vi "Host Processing (SubVI).vi"(4 "Channel Data":cluster{"AI":T1, "DI":T5, "DO":T5, "Async":T8}={"AI"={"Interface"="AIO", "Interface Data"={"Command"="Configure", "SubCmd"="AI", "Data"=[{"Channel"="Mod1/ai0", "Min Value"=-5.0, "Max Value"=5.0, "Type"="Voltage", "Terminal Configure"=10083, "Dynamic"=0, "Dyn Type"="", "Data"=[], "File Name"="", "Column"=0, "Frequency"=0.0}, {"Channel"="Mod1/ai1", "Min Value"=-5.0, "Max Value"=5.0, "Type"="Voltage", "Terminal Configure"=10083, "Dynamic"=0, "Dyn Type"="", "Data"=[], "File Name"="", "Column"=0, "Frequency"=0.0}], "Timing"={"samples per channel"=4, "sample mode"=10123, "rate"=2.0}}}, "DI"={"Interface"="DIO", "Interface Data"={"Command"="Configure", "SubCmd"="DI", "Frequency"=20, "Data"=[{"Channel"="Mod2/port0/line0", "Data"=[], "Identification Name"=""}, {"Channel"="Mod2/port0/line1", "Data"=[], "Identification Name"=""}, {"Channel"="Mod2/port0/line2", "Data"=[], "Identification Name"=""}, {"Channel"="Mod2/port0/line3", "Data"=[], "Identification Name"=""}]}}, "DO"={"Interface"="DIO", "Interface Data"={"Command"="Configure", "SubCmd"="DO", "Frequency"=20, "Data"=[{"Channel"="Mod2/port0/line0", "Data"=[], "Identification Name"=""}, {"Channel"="Mod2/port0/line1", "Data"=[], "Identification Name"=""}, {"Channel"="Mod2/port0/line2", "Data"=[], "Identification Name"=""}, {"Channel"="Mod2/port0/line3", "Data"=[], "Identification Name"=""}]}}, "Async"={"Interface"="Async", "Interface Data"={"Command"="Configure", "SubCmd"="Async", "Data"=[{"Port"="com2", "Minor Frame Freq"=20, "Minor Frame Count"=1, "Frame Info"=[{"Frame ID"=1, "Message Info"=[{"Message"=[1, 2, 3, 4], "Message Name"="m1"}]}], "Sensor Type"=0, "OIM Address"=0}]}}} {"Async"."Interface Data"."Data"."Minor Frame Count" min=5 max=8 step=1; "AI"."Interface Data"."Timing"."sample mode" items=["Finite Samples"=10178, "Continuous Samples"=10123, "Hardware Timed Single Point"=12522]}, 5 "Serial Data":T13[](array[typedef]), 6 "Operation":T14(ring), 7 "DO Data":cluster{"Channel":string[], "Data":u8[]}={"Channel"=["Mod2/port1/line0", "Mod2/port1/line1", "Mod2/port1/line2", "Mod2/port1/line3"], "Data"=[0, 0, 0, 0]}, 8 "error in":errorcluster, 9 "connection ID in":refnum<k5>, 10 "queue in":refnum<queue>, 11 "IP":string) -> (0 "error out":errorcluster, 1 "connection ID":refnum<k5>, 2 "Queue out":refnum<queue>, 3 "data out":string)   [LabVIEW 2021]
uses:
  Async Serial/Controls/Async Message Info Cluster.ctl
  Async Serial/Controls/Async Update Cluster.ctl
  407f0374-129d-499a-9c6e-116d754379dc.vi
  Digital Output/SubVIs/Digital Dynamic Cluster.ctl
  Digital Output/Controls/DIO Interface Data.ctl
  Digital Output/Controls/DIO Configuration cluster.ctl
  Async Serial/Controls/Async Frame Info Cluster.ctl
  Async Serial/Controls/Async Serial Configuration Cluster.ctl
  Async Interface Data Cluster.ctl
  Async JSON Cluster.ctl
  Analog Output/Controls/AO Timing Cluster.ctl
  Analog Output/Controls/AO Channel Configuration Cluster.ctl
  Analog Output/Controls/AO Interface Data Cluster.ctl
  Analog Output/Controls/AO JSON Data Cluster.ctl
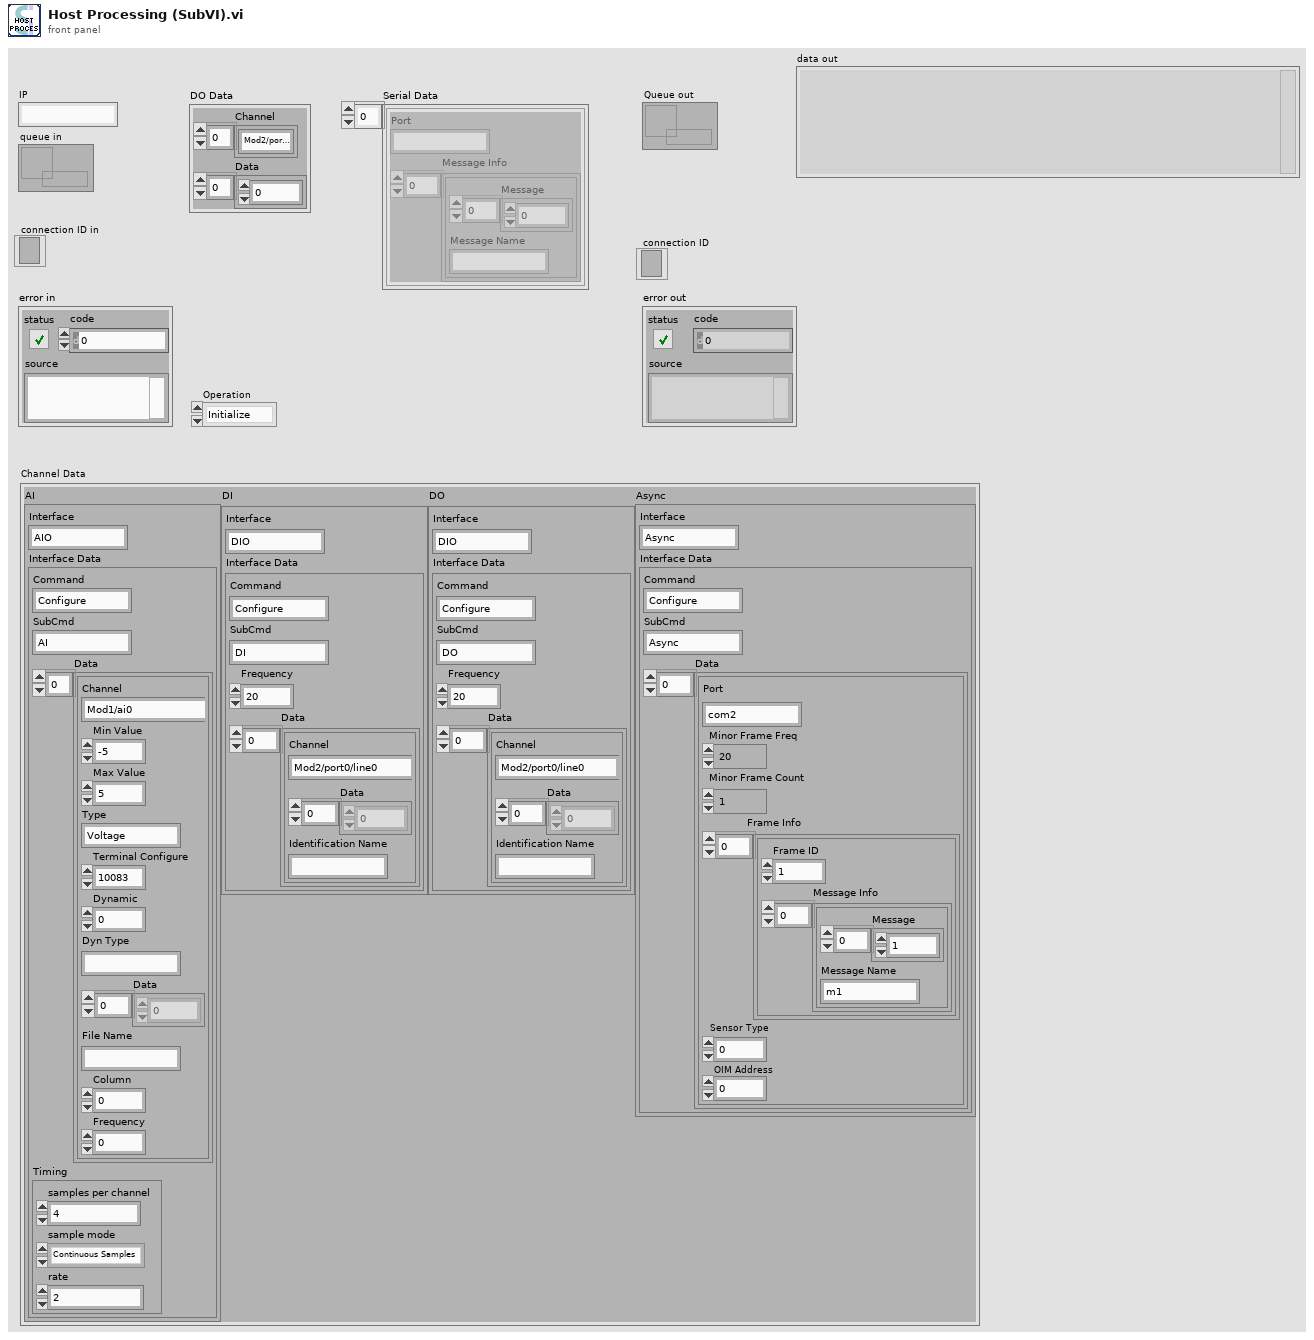
[diagram p1: front panel]
types:
  T1 = typedef "AO JSON Data Cluster.ctl" = cluster{"Interface":string, "Interface Data":T2}
  T2 = typedef "AO Interface Data Cluster.ctl" = cluster{"Command":string, "SubCmd":string, "Data":T3[], "Timing":T4}
  T3 = typedef "AO Channel Configuration Cluster.ctl" = cluster{"Channel":string, "Min Value":dbl, "Max Value":dbl, "Type":string, "Terminal Configure":u16, "Dynamic":u8, "Dyn Type":string, "Data":dbl[], "File Name":string, "Column":i32, "Frequency":dbl}
  T4 = typedef "AO Timing Cluster.ctl" = cluster{"samples per channel":i32, "sample mode":i32, "rate":dbl}
  T5 = typedef "DIO Configuration cluster.ctl" = cluster{"Interface":string, "Interface Data":T6}
  T6 = typedef "DIO Interface Data.ctl" = cluster{"Command":string, "SubCmd":string, "Frequency":u16, "Data":T7[]}
  T7 = typedef "Digital Dynamic Cluster.ctl" = cluster{"Channel":string, "Data":u8[], "Identification Name":string}
  T8 = typedef "Async JSON Cluster.ctl" = cluster{"Interface":string, "Interface Data":T9}
  T9 = typedef "Async Interface Data Cluster.ctl" = cluster{"Command":string, "SubCmd":string, "Data":T10[]}
  T10 = typedef "Async Serial Configuration Cluster.ctl" = cluster{"Port":string, "Minor Frame Freq":u16, "Minor Frame Count":u16, "Frame Info":T11[], "Sensor Type":u16, "OIM Address":u16}
  T11 = typedef "Async Frame Info Cluster.ctl" = cluster{"Frame ID":u16, "Message Info":T12[]}
  T12 = typedef "Async Message Info Cluster.ctl" = cluster{"Message":u8[], "Message Name":string}
  T13 = typedef "Async Update Cluster.ctl" = cluster{"Port":string, "Message Info":T12[]}
  T14 = enum16{"Initialize", "Read", "Update DO", "Update Serial", "Exit"}
  T15 = enum16{"Standard", "Buffered", "CRLF", "Immediate"}
  T16 = enum16{"big-endian, network order", "native, host order", "little-endian"}
  T17 = cluster{"Interface":string, "Interface Data":cluster{"Command":string, "SubCmd":string, "Channel":string[], "Data":u8[]}}
  T18 = cluster{"Interface":string, "Interface Data":cluster{"Command":string, "SubCmd":string, "Data":T13[]}}
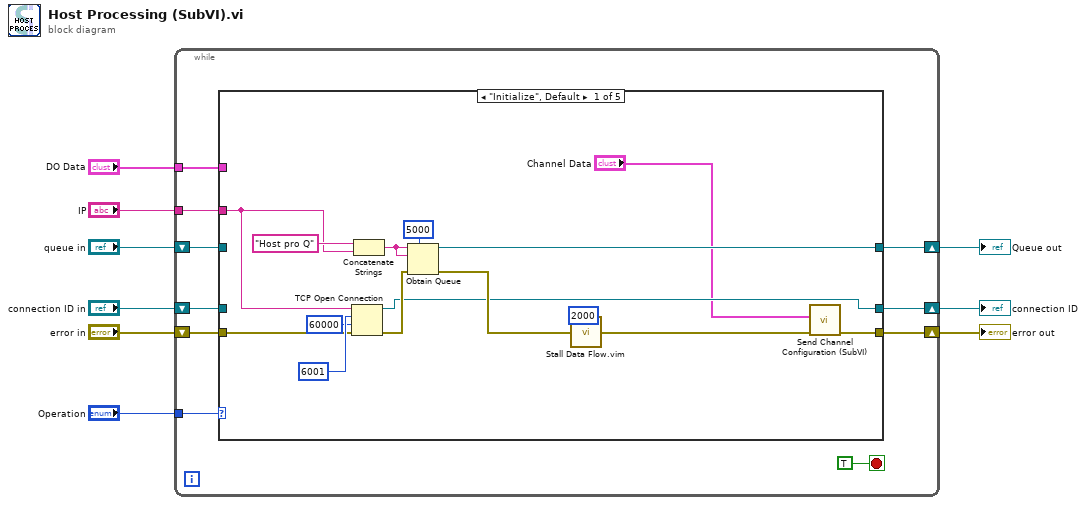
[diagram p0: block diagram]
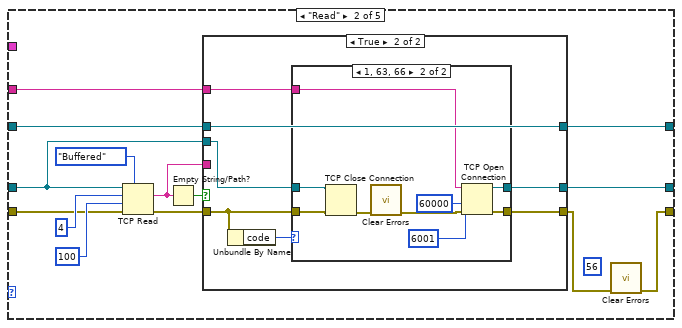
[diagram p2: hidden frame]
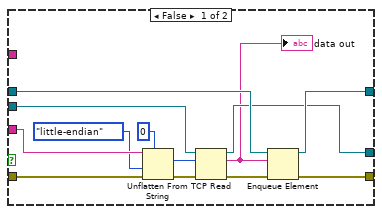
[diagram p3: hidden frame]
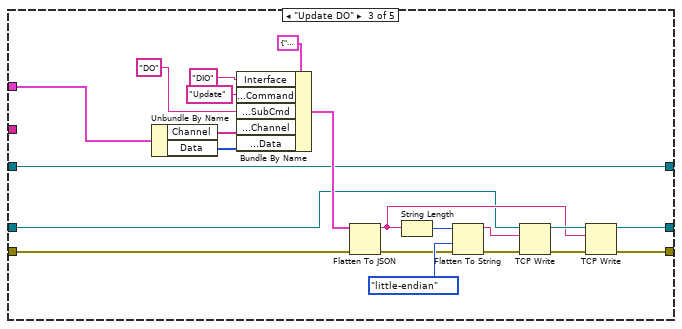
[diagram p5: hidden frame]
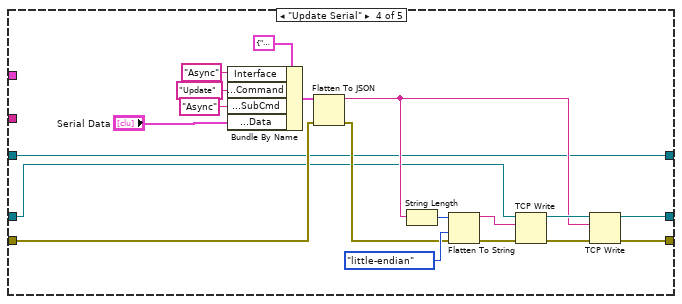
[diagram p6: hidden frame]
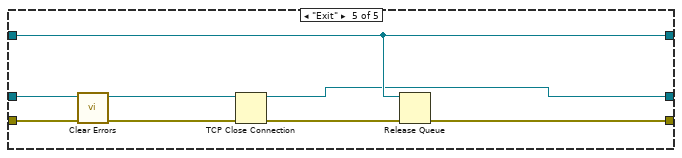
[diagram p7: hidden frame]
diagram:
  n1 = while {
    tunnel: "Operation" -> [w18]
    shift-right: [w17] -> w6
    shift-left: "error in" -> [w16]
    shift-right: [w15] -> w8
    shift-left: "queue in" -> [w14]
    shift-right: [w13] -> w3
    shift-left: "connection ID in" -> [w12]
    tunnel: "IP" -> [w11]
    tunnel: "DO Data" -> [w10]
    stop <- TRUE stop-if-true
    n2 = case shown="\"Initialize\", Default" w18 {
      tunnel: [w26 w36 w83 w103 w123] -> w17
      tunnel: w16 -> [w33 w42 w84 w106 w126]
      tunnel: [w28 w38 w80 w101 w121] -> w15
      tunnel: w14 -> [_ w41 w80 w101 w121]
      tunnel: [w21 w39 w82 w102 w120] -> w13
      tunnel: w12 -> [_ w40 w81 w104 w125]
      tunnel: w11 -> [w27 w35 _ _ _]
      tunnel: w10 -> [_ _ w85 _ _]
      frame "Initialize", Default {
        n3 = TCP Open Connection(address=w27, remote port or service name=u16 6001 ("local port"), timeout ms (60000)=60000, error in (no error)=w33) -> (connection ID=w21:refnum<k5>, error out=w29:errorcluster)  [unwired: 1 in]
        n4 = Concatenate Strings("Host pro Q" ("name (unnamed)"), w27) -> (w30:string)
        n5 = Obtain Queue(max queue size (-1, unlimited)=5000, name (unnamed)=w30, element data type=w30, error in (no error)=w29) -> (queue out=w28:refnum<queue>, error out=w24:errorcluster)  [unwired: 1 in, 1 out]
        n6 = call "Stall Data Flow.vim"("value in"=w24, "milliseconds to wait"=u32 2000) -> ("value out"=w23:errorcluster)  [unwired: 1 out]
        n7 = call "Send Channel Configuration (SubVI).vi"("error in"=w23, 10:"Channel Data") -> ("error out"=w26:errorcluster)  [unwired: 8 in, 1 out]
      }
      frame "Read" {
        (unwired) 56 ("specific error code to clear (0: all)")
        n8 = TCP Read(connection ID=w40, bytes to read=4, error in (no error)=w42, 7:T15."Buffered" ("mode (standard)"), 9:100 ("timeout ms (25000)")) -> (data out=w43:string, error out=w46:errorcluster)  [unwired: 1 out]
        n9 = Empty String/Path?(string/path=w43) -> (empty?=w47:bool)
        n10 = case shown="True" w47 {
          tunnel: w43 -> [w56 _]
          tunnel: w40 -> [w60 w66]
          tunnel: w46 -> [w58 w64]
          tunnel: w41 -> [w54 w68]
          tunnel: [w52 w63] -> w37
          tunnel: [w50 w62] -> w39
          tunnel: [w51 w68] -> w38
          tunnel: w35 -> [_ w65]
          frame False {
            n11 = Unflatten From String(type=0, binary string=w56, byte order (0:big-endian, network order)=T16."little-endian", error in (no error)=w58) -> (value=w59:i32, error out=w57:errorcluster)  [unwired: 1 in, 1 out]
            n12 = TCP Read(connection ID=w60, bytes to read=w59, error in (no error)=w57) -> (connection ID out=w50:refnum<k5>, data out=w49:string, error out=w53:errorcluster)  [unwired: 2 in]
            "data out" <- w49
            n13 = Enqueue Element(queue=w54, element=w49, error in (no error)=w53) -> (queue out=w51:refnum<queue>, error out=w52:errorcluster)  [unwired: 1 in, 1 out]
          }
          frame True {
            n14 = Unbundle By Name(w64) -> ("code"=w67:i32)
            n15 = case shown="1, 63, 66" w67 {
              tunnel: w64 -> [w69 w79]
              tunnel: w66 -> [w70 w78]
              tunnel: w65 -> [_ w74]
              tunnel: [w69 w72] -> w63
              tunnel: [w70 w71] -> w62
              frame 0, Default {
              }
              frame 1, 63, 66 {
                n16 = TCP Close Connection(connection ID=w78, error in (no error)=w79) -> (error out=w77:errorcluster)  [unwired: 1 in, 1 out]
                n17 = call <vilib>:"Clear Errors.vi"("error in (no error)"=w77) -> ("error out"=w73:errorcluster)  [unwired: 5 in, 1 out]
                n18 = TCP Open Connection(address=w74, remote port or service name=u16 6001 ("local port"), timeout ms (60000)=60000, error in (no error)=w73) -> (connection ID=w71:refnum<k5>, error out=w72:errorcluster)  [unwired: 1 in]
              }
            }
          }
        }
        n19 = call <vilib>:"Clear Errors.vi"("error in (no error)"=w37) -> ("error out"=w36:errorcluster)  [unwired: 5 in, 1 out]
      }
      frame "Update DO" {
        n20 = Unbundle By Name(w85) -> ("Channel"=w89:string[], "Data"=w88:u8[])
        n21 = Bundle By Name(cluster=T17 {"Interface"="", "Interface Data"={"Command"="", "SubCmd"="", "Channel"=[], "Data"=[]}}, "Interface"="DIO", "Interface Data.Command"="Update", "Interface Data.SubCmd"="DO" ("Interface Data.Sub Cmd"), "Interface Data.Channel"=w89, "Interface Data.Data"=w88) -> (w96:T17)
        n22 = Flatten To JSON(anything=w96, error in (no error)=w84) -> (JSON string=w87:string, 11:w86:errorcluster)  [unwired: 1 in]
        n23 = String Length(string=w87) -> (length=w93:i32)
        n24 = Flatten To String(anything=w93, byte order (0:big-endian, network order)=T16."little-endian", error in (no error)=w86) -> (data string=w91:string, error out=w90:errorcluster)  [unwired: 1 in, 1 out]
        n25 = TCP Write(connection ID=w81, data in=w91, error in (no error)=w90) -> (connection ID out=w95:refnum<k5>, error out=w94:errorcluster)  [unwired: 1 in, 1 out]
        n26 = TCP Write(connection ID=w95, data in=w87, error in (no error)=w94) -> (connection ID out=w82:refnum<k5>, error out=w83:errorcluster)  [unwired: 1 in, 1 out]
      }
      frame "Update Serial" {
        n27 = Bundle By Name(cluster=T18 {"Interface"="", "Interface Data"={"Command"="", "SubCmd"="", "Data"=[]}}, "Interface"="Async", "Interface Data.Command"="Update", "Interface Data.SubCmd"="Async", "Interface Data.Data"="Serial Data") -> (w110:T18)
        n28 = Flatten To JSON(anything=w110, error in (no error)=w106) -> (JSON string=w109:string, 11:w105:errorcluster)  [unwired: 1 in]
        n29 = String Length(string=w109) -> (length=w117:i32)
        n30 = Flatten To String(anything=w117, byte order (0:big-endian, network order)=T16."little-endian", error in (no error)=w105) -> (data string=w115:string, error out=w114:errorcluster)  [unwired: 1 in, 1 out]
        n31 = TCP Write(connection ID=w104, data in=w115, error in (no error)=w114) -> (connection ID out=w119:refnum<k5>, error out=w118:errorcluster)  [unwired: 1 in, 1 out]
        n32 = TCP Write(connection ID=w119, data in=w109, error in (no error)=w118) -> (connection ID out=w102:refnum<k5>, error out=w103:errorcluster)  [unwired: 1 in, 1 out]
      }
      frame "Exit" {
        n33 = call <vilib>:"Clear Errors.vi"("error in (no error)"=w126) -> ("error out"=w122:errorcluster)  [unwired: 5 in, 1 out]
        n34 = TCP Close Connection(connection ID=w125, error in (no error)=w122) -> (connection ID out=w120:refnum<k5>, error out=w124:errorcluster)  [unwired: 1 in]
        n35 = Release Queue(queue=w121, error in (no error)=w124) -> (error out=w123:errorcluster)  [unwired: 1 in, 2 out]
      }
    }
  }
  "Queue out" <- w8
  "error out" <- w6
  "connection ID" <- w3
